vi "Generatore di numeri primi versione 9.0.vi"(0 "Numero di numeri\nprimi desiderati":i32=20000, 1 "stop":bool) -> (2 "Numero\nprimo":i32[](array[numeric]), 3 "Numero primo\ncorrente":i32, 4 "Tempo trascorso":dbl)   [LabVIEW 2012]
uses:
  <vilib>/Utility/file.llb/Write To Spreadsheet File (I64).vi
panel:
  out "Waveform Chart":i32(graph)
  # "Numeri primi"
  # "Dopo aver fatto girare il programma,\ninserisci l'indice del numero primo desiderato"
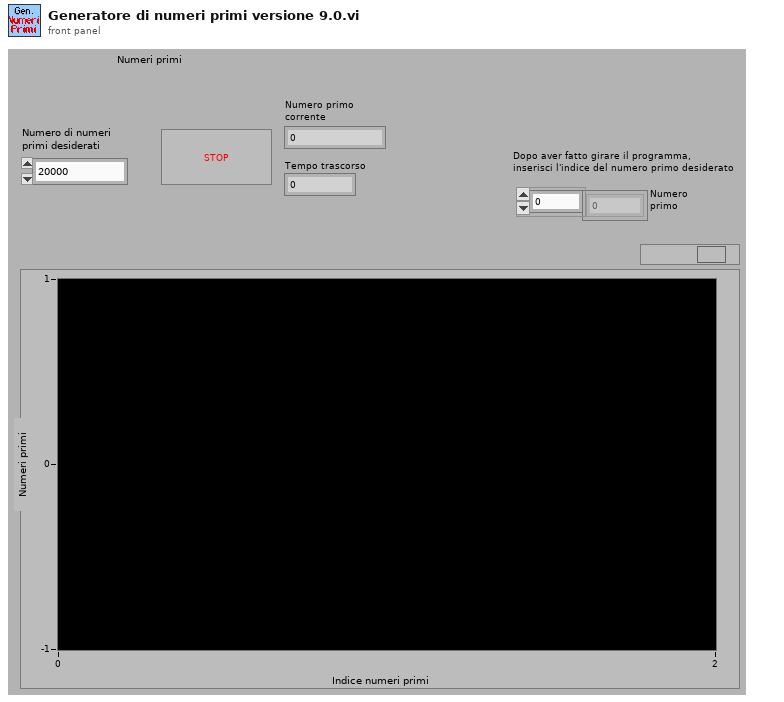
[diagram p1: front panel]
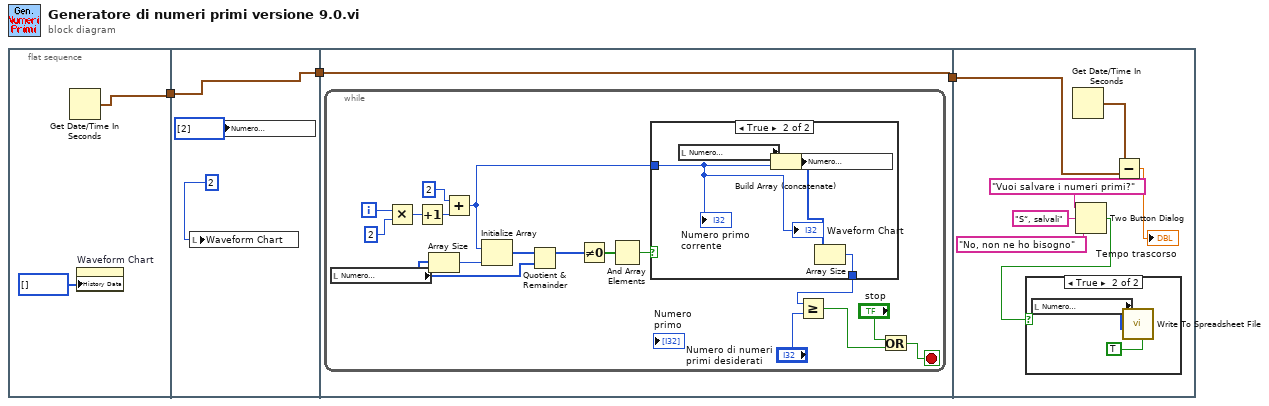
[diagram p0: block diagram]
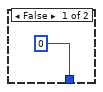
[diagram p2: hidden frame]
diagram:
  n1 = flat-sequence {
    tunnel: [w4] -> w3
    tunnel: w3 -> [w6]
    tunnel: [w6] -> w2
    tunnel: w2 -> [w9]
    tunnel: [w9] -> w1
    tunnel: w1 -> [w37]
    frame #0 {
      n2 = Get Date/Time In Seconds() -> (seconds since 1Jan1904=w4:timestamp)
      n3 = property on="Waveform Chart" class="WFChart (strict)"("History Data"=i32[] []) -> ()  [unwired: 2 in, 2 out]
    }
    frame #1 {
      n4 = local write "Waveform Chart"(2 ("Numeric")) -> ()
      n5 = local write "Numero\nprimo"(i32[] [2] ("Primes")) -> ()
    }
    frame #2 {
      n6 = while {
        i -> [w11]
        stop <- w17 stop-if-true
        n7 = local read "Numero\nprimo"() -> (w25:i32[])
        n8 = Multiply(x=w11, y=2) -> (x*y=w12:i32)
        n9 = Increment(x=w12) -> (x+1=w10:i32)
        n10 = Array Size(array=w25) -> (size(s)=w26:i32)
        n11 = Add(x=2, y=w10) -> (x+y=w20:i32)
        n12 = Initialize Array(w20, w26) -> (w24:i32[])
        n13 = Quotient & Remainder(x=w24, y=w25) -> (x-y*floor(x/y)=w23:i32[])  [unwired: 1 out]
        n14 = Not Equal To 0?(x=w23) -> (x != 0?=w22:bool[])
        n15 = And Array Elements(Boolean array=w22) -> (logical AND=w21:bool)
        n16 = case shown="True" w21 {
          tunnel: w20 -> [_ w30]
          tunnel: [0 w28] -> w16
          frame False {
          }
          frame True {
            n17 = local read "Numero\nprimo"() -> (w31:i32[])
            n18 = Build Array (concatenate)(w31, w30) -> (w29:i32[])
            n19 = local write "Numero\nprimo"(w29) -> ()
            n20 = Array Size(array=w29) -> (size(s)=w28:i32)
            "Numero primo\ncorrente" <- w30
            "Waveform Chart" <- w30
          }
        }
        n21 = Greater Or Equal?(x=w16, y="Numero di numeri\nprimi desiderati") -> (x >= y?=w14:bool)
        n22 = Or(x="stop", y=w14) -> (x .or. y?=w17:bool)
      }
    }
    frame #3 {
      n23 = Get Date/Time In Seconds() -> (seconds since 1Jan1904=w38:timestamp)
      n24 = Two Button Dialog(message="Vuoi salvare i numeri primi?", 1:"No, non ne ho bisogno" ("F button name (\"Cancel\")"), 2:"S“, salvali" ("T button name (\"OK\")")) -> (T button?=w35:bool)
      n25 = case shown="True" w35 {
        frame False {
        }
        frame True {
          n26 = local read "Numero\nprimo"() -> (w40:i32[])
          n27 = call-poly <vilib>:"Write To Spreadsheet File.vi"("transpose? (no:F)"=TRUE, "1D data"=w40) -> ()  [unwired: 6 in, 1 out]
        }
      }
      n28 = Subtract(x=w38, y=w37) -> (x-y=→"Tempo trascorso":dbl)
    }
  }
